vi "cal_main_bool_const_pos.vi"(1 "Disable String":string="OFF", 5 "Main Node BD Position":cluster{"Left":i32, "Top":i32}, 11 "error in (no error)":errorcluster) -> (6 "Enable Constant Position":cluster{"Left":i32, "Top":i32}, 8 "Disable Constant Position":cluster{"Left":i32, "Top":i32}, 15 "error out":errorcluster)   [LabVIEW 2018]
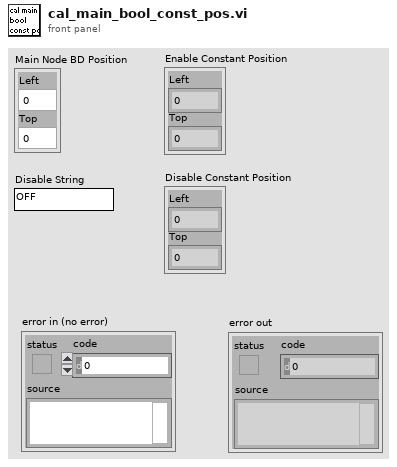
[diagram p1: front panel]
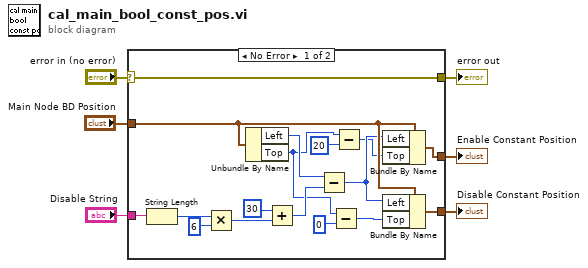
[diagram p0: block diagram]
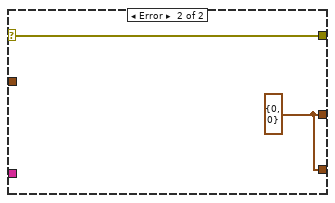
[diagram p2: hidden frame]
diagram:
  n1 = case shown="No Error" "error in (no error)" {
    selector: "error in (no error)" -> [w8 w24]
    tunnel: "Main Node BD Position" -> [w23 _]
    tunnel: "Disable String" -> [w20 _]
    tunnel: [w14 w25] -> w4
    tunnel: [w13 w25] -> w3
    tunnel: [w8 w24] -> w1
    frame No Error {
      n2 = String Length(string=w20) -> (length=w17:i32)
      n3 = Multiply(x=w17, y=6) -> (x*y=w19:i32)
      n4 = Unbundle By Name(w23) -> ("Left"=w9:i32, "Top"=w7:i32)
      n5 = Add(x=30, y=w19) -> (x+y=w21:i32)
      n6 = Subtract(x=w9, y=w21) -> (x-y=w15:i32)
      n7 = Subtract(x=w7, y=0) -> (x-y=w16:i32)
      n8 = Subtract(x=w7, y=20) -> (x-y=w12:i32)
      n9 = Bundle By Name(cluster=w23, "Left"=w15, "Top"=w12) -> (w13:cluster{"Left":i32, "Top":i32})
      n10 = Bundle By Name(cluster=w23, "Left"=w15, "Top"=w16) -> (w14:cluster{"Left":i32, "Top":i32})
    }
    frame Error {
      w25 = cluster{"Left":i32, "Top":i32} {"Left"=0, "Top"=0} ("Main Node BD Position")
    }
  }
  "Disable Constant Position" <- w4
  "Enable Constant Position" <- w3
  "error out" <- w1
